vi "VCS Read Position Marker Captured Position.vi"(0 "axis in":cluster{"keyHandle":u32, "nodeId":u16}={"keyHandle"=0, "nodeId"=1}, 7 "counterIndex":u16, 11 "error in (no error)":errorcluster) -> (4 "axis out":cluster{"keyHandle":u32, "nodeId":u16}={"keyHandle"=0, "nodeId"=1}, 10 "capturedPosition":i32, 15 "error out":errorcluster)   [LabVIEW 2019, in "maxonEPOS.lvlib"]
doc: "<B>VCS_ReadPositionMarkerCapturedPosition</B> returns the last captured position."
uses:
  Examples/maxonEPOS.lvlib
  Resources/EposCmd.dll
  Resources/EposCmd64.dll
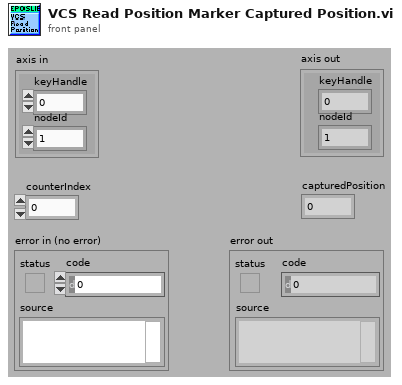
[diagram p1: front panel]
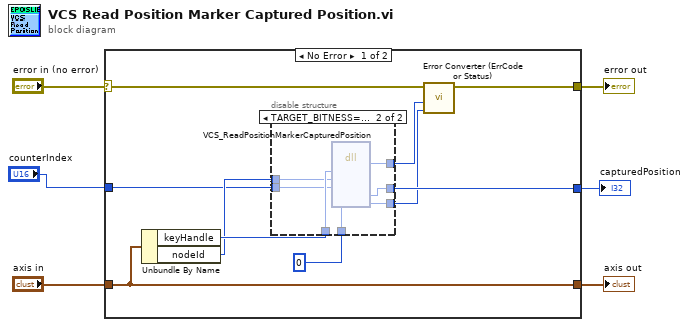
[diagram p0: block diagram]
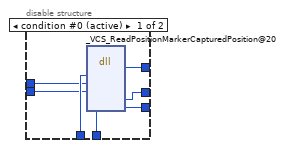
[diagram p2: hidden frame]
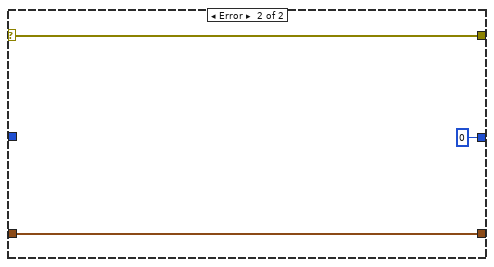
[diagram p3: hidden frame]
diagram:
  n1 = case shown="No Error" "error in (no error)" {
    selector: "error in (no error)" -> [w14 w32]
    tunnel: "axis in" -> [w16 w33]
    tunnel: [w16 w33] -> w5
    tunnel: [w15 w32] -> w4
    tunnel: "counterIndex" -> [w10 _]
    tunnel: [w9 0 ("pCapturedPosition")] -> w1
    frame No Error {
      n2 = Unbundle By Name(w16) -> ("keyHandle"=w13:u32, "nodeId"=w12:u16)
      n3 = disable-structure shown="TARGET_BITNESS==64" {
        disable-tunnel: w13 -> [w23 w30]
        disable-tunnel: w12 -> [w22 w29]
        disable-tunnel: u32 0 ("pErrorCode") -> [w21 w28]
        disable-tunnel: w10 -> [w20 w27]
        disable-tunnel: [w19 w26] -> w9
        disable-tunnel: [w18 w25] -> w8
        disable-tunnel: [w17 w24] -> w7
        frame condition #0 (active) {
          n4 = dll-call lib="C:/workspace/project/scancon/sw/SSI_Tool/InstrumentsInterfaces/Motordriver/maxon EPOS/Resources/EposCmd.*" fn="_VCS_ReadPositionMarkerCapturedPosition@20"("KeyHandle"=w23, "NodeId"=w22, "CounterIndex"=w20, "pErrorCode"=w21) -> (w18:i32, "pCapturedPosition"=w19:i32, "pErrorCode"=w17:u32)  [unwired: 7 in, 2 out]
        }
        frame condition #1 {
          n5 = dll-call lib="C:/setup/Resources/EposCmd64.*" fn="VCS_ReadPositionMarkerCapturedPosition" ("EposCmd.dll:_VCS_ReadPositionMarkerCapturedPosition@20")("KeyHandle"=w30, "NodeId"=w29, "CounterIndex"=w27, "pErrorCode"=w28) -> ("Rückgabetyp"=w25:i32, "pCapturedPosition"=w26:i32, "pErrorCode"=w24:u32)  [unwired: 7 in, 2 out]
        }
      }
      n6 = call "Error Converter (ErrCode or Status).vi"("error code"=w7, "return type"=w8, "error in (no error)"=w14) -> ("error out"=w15:errorcluster)  [unwired: 7 in]
    }
    frame Error {
    }
  }
  "capturedPosition" <- w1
  "error out" <- w4
  "axis out" <- w5
